vi "test_MonoOpenAndClose.vi"(6 "Delay between send and receive [ms]":i32=100, 7 "Test should pass":bool=TRUE, 8 "error in":errorcluster, 9 "tear down connection":bool=TRUE, 10 "set-up a connection":bool=TRUE, 11 "device selection":enum16{"monochromator", "CCD", "SCD"}(ring)) -> (0 "error out":errorcluster, 1 "log-file path":path)   [LabVIEW 2023]
uses:
  Classes/Mono/Monochromator.lvclass
  <vilib>/addons/_JKI Toolkits/Caraya/classes/Assert/Assert Equal Value and Type_Variant.vi
  <vilib>/addons/_JKI Toolkits/Caraya/classes/Assert/Assert Not Error.vi
  <vilib>/addons/_JKI Toolkits/Caraya/classes/Test/Test.lvclass
  <vilib>/addons/_JKI Toolkits/Caraya/classes/Assert/Assert.lvclass
  <vilib>/Hampel Software Engineering/HSE Logger/hse-logger.lvlib
panel:
  # "Connector Pane"
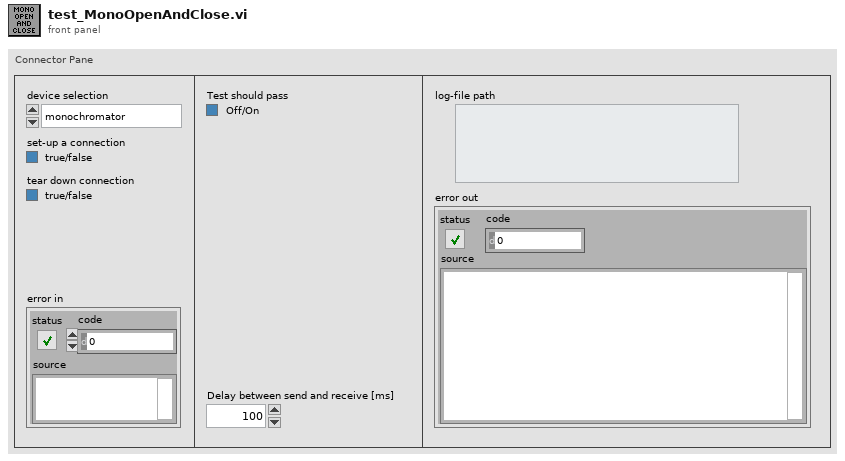
[diagram p1: front panel]
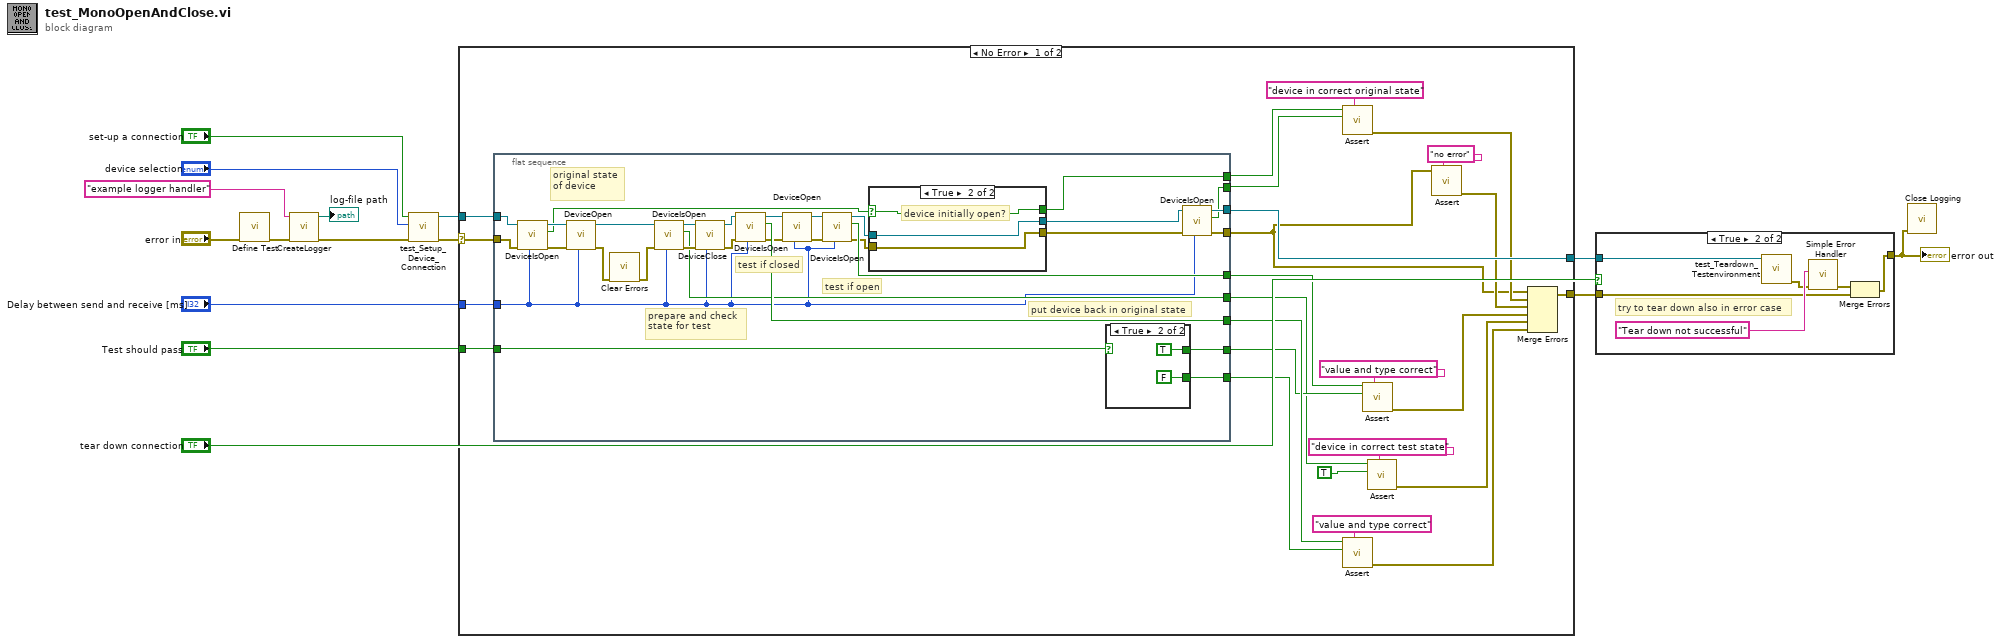
[diagram p0: block diagram]
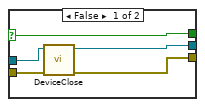
[diagram p2: hidden frame]
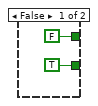
[diagram p3: hidden frame]
diagram:
  n1 = call <vilib>:"Define Test.vi"("error in (no error)"="error in") -> ("error out"=w6:errorcluster)  [unwired: 9 in, 1 out]
  n2 = call "CreateLogger.vi"("error in (no error)"=w6, "Handler Name"="example logger handler") -> ("error out"=w4:errorcluster, "log-file path"=→"log-file path":path)  [unwired: 8 in]
  n3 = call "test_Setup_Device_Connection.vi"("error in (no error)"=w4, "device selection"="device selection", "set-up a connection"="set-up a connection") -> ("error out"=w7:errorcluster, "Monochromator.lvclass"=w10:refnum<class "Monochromator.lvclass">)  [unwired: 5 in, 2 out]
  n4 = case shown="No Error" w7 {
    selector: w7 -> [w17 w85]
    tunnel: "Test should pass" -> [w36 _]
    tunnel: [w35 w84] -> w11
    tunnel: w10 -> [w24 w84]
    tunnel: [w18 w85] -> w8
    tunnel: "Delay between send and receive [ms]" -> [w16 _]
    frame No Error {
      n5 = flat-sequence {
        tunnel: w17 -> [w70]
        tunnel: [w46] -> w19
        tunnel: w36 -> [w71]
        tunnel: [w50] -> w35
        tunnel: [w63] -> w34
        tunnel: [w62] -> w33
        tunnel: [w61] -> w32
        tunnel: [w60] -> w31
        tunnel: [w59] -> w29
        tunnel: [w52] -> w26
        tunnel: [w49] -> w25
        tunnel: w24 -> [w42]
        tunnel: w16 -> [w41]
        frame #0 {
          # "put device back in original state"
          # "test if open"
          # "test if closed"
          # "original state of device"
          # "prepare and check state for test"
          n6 = call-dynamic "DeviceIsOpen.vi"("Delay between send and receive [ms]"=w41, "error in (no error)"=w70, "Monochromator in"=w42) -> ("error out"=w45:errorcluster, "device is open?"=w58:bool, "Monochromator out"=w69:refnum<class "Monochromator.lvclass">)  [unwired: 5 in, 1 out]
          n7 = call-dynamic "DeviceOpen.vi"("Delay between send and receive [ms]"=w41, "error in (no error)"=w45, "Monochromator in"=w69) -> ("error out"=w44:errorcluster, "Monochromator out"=w68:refnum<class "Monochromator.lvclass">)  [unwired: 5 in, 2 out]
          n8 = call <vilib>:"Clear Errors.vi"("error in (no error)"=w44) -> ("error out"=w43:errorcluster)  [unwired: 5 in, 1 out]
          n9 = call-dynamic "DeviceIsOpen.vi"("Delay between send and receive [ms]"=w41, "error in (no error)"=w43, "Monochromator in"=w68) -> ("error out"=w64:errorcluster, "device is open?"=w59:bool, "Monochromator out"=w67:refnum<class "Monochromator.lvclass">)  [unwired: 5 in, 1 out]
          n10 = call-dynamic "DeviceClose.vi"("Delay between send and receive [ms]"=w41, "error in (no error)"=w64, "Monochromator in"=w67) -> ("error out"=w65:errorcluster, "Monochromator out"=w66:refnum<class "Monochromator.lvclass">)  [unwired: 4 in, 3 out]
          n11 = call-dynamic "DeviceIsOpen.vi"("Delay between send and receive [ms]"=w41, "error in (no error)"=w65, "Monochromator in"=w66) -> ("error out"=w54:errorcluster, "device is open?"=w63:bool, "Monochromator out"=w56:refnum<class "Monochromator.lvclass">)  [unwired: 5 in, 1 out]
          n12 = call-dynamic "DeviceOpen.vi"("Delay between send and receive [ms]"=w41, "error in (no error)"=w54, "Monochromator in"=w56) -> ("error out"=w53:errorcluster, "Monochromator out"=w55:refnum<class "Monochromator.lvclass">)  [unwired: 5 in, 2 out]
          n13 = call-dynamic "DeviceIsOpen.vi"("Delay between send and receive [ms]"=w41, "error in (no error)"=w53, "Monochromator in"=w55) -> ("error out"=w48:errorcluster, "device is open?"=w61:bool, "Monochromator out"=w57:refnum<class "Monochromator.lvclass">)  [unwired: 5 in, 1 out]
          n14 = case shown="True" w58 {
            selector: w58 -> [w74 w77]
            tunnel: w57 -> [w76 w79]
            tunnel: [w75 w79] -> w51
            tunnel: [w74 w77] -> w52
            tunnel: w48 -> [w73 w78]
            tunnel: [w72 w78] -> w47
            frame False {
              n15 = call-dynamic "DeviceClose.vi"("error in (no error)"=w73, "Monochromator in"=w76) -> ("error out"=w72:errorcluster, "Monochromator out"=w75:refnum<class "Monochromator.lvclass">)  [unwired: 5 in, 3 out]
            }
            frame True {
              # "device initially open?"
            }
          }
          n16 = case shown="True" w71 {
            tunnel: [TRUE ("device is open?") FALSE ("device is open?")] -> w62
            tunnel: [FALSE ("device is open?") TRUE ("device is open?")] -> w60
            frame False {
            }
            frame True {
            }
          }
          n17 = call-dynamic "DeviceIsOpen.vi"("Delay between send and receive [ms]"=w41, "error in (no error)"=w47, "Monochromator in"=w51) -> ("error out"=w46:errorcluster, "device is open?"=w49:bool, "Monochromator out"=w50:refnum<class "Monochromator.lvclass">)  [unwired: 5 in, 1 out]
        }
      }
      n18 = call-poly <vilib>:"Assert.vi"("Label"="device in correct original state" ("Label (VI Title)"), "Y"=w25, "X"=w26) -> ("error out"=w20:errorcluster)  [unwired: 7 in, 1 out]
      n19 = call-poly <vilib>:"Assert.vi"("Label"="value and type correct" ("Label (VI Title)"), "Y"=w33, "X"=w34) -> ("error out"=w22:errorcluster)  [unwired: 7 in, 1 out]
      n20 = call-poly <vilib>:"Assert.vi"("Label"="value and type correct" ("Label (VI Title)"), "Y"=w31, "X"=w32) -> ("error out"=w39:errorcluster)  [unwired: 7 in, 1 out]
      n21 = call-poly <vilib>:"Assert.vi"("Label"="device in correct test state" ("Label (VI Title)"), "Y"=TRUE ("device is open?"), "X"=w29) -> ("error out"=w23:errorcluster)  [unwired: 7 in, 1 out]
      n22 = call-poly <vilib>:"Assert.vi"("Label"="no error" ("Label (VI Title)"), "Not Error?"=w19) -> ("error out"=w21:errorcluster)  [unwired: 8 in, 1 out]
      n23 = Merge Errors(w19, w20, w21, w39, w23, w22) -> (w18:errorcluster)
    }
    frame Error {
    }
  }
  n24 = case shown="True" "tear down connection" {
    tunnel: w11 -> [_ w91]
    tunnel: [w86 w87] -> w2
    tunnel: w8 -> [w86 w88]
    frame False {
    }
    frame True {
      # "try to tear down also in error case"
      n25 = call "test_Teardown_Testenvironment.vi"("GenericDevice.lvclass"=w91) -> ("error out"=w90:errorcluster)  [unwired: 9 in, 1 out]
      n26 = call <vilib>:"Simple Error Handler.vi"("error source (\" \")"="Tear down not successful" ("error source (\" \")"), "error in (no error)"=w90) -> ("error out"=w89:errorcluster)  [unwired: 3 in, 4 out]
      n27 = Merge Errors(w89, w88) -> (w87:errorcluster)
    }
  }
  "error out" <- w2
  n28 = call <vilib>:"Close Logging.vi"("error in"=w2) -> ()  [unwired: 10 in, 1 out]
